vi "Current_Calib_Filenames.vi"(3 "Calib Filename":path[](array[path]), 4 "Channel Numbers":i16[](array[numeric]) min=0 max=7, 5 "Mode":T1) -> (0 "Calib Filename Out":path[](array[path]), 1 "Channel Numbers Out":i16[](array[numeric]) min=0 max=7)   [LabVIEW 2010]
uses:
  Controls/App_Global.ctl
  Globals/Constants_global.vi
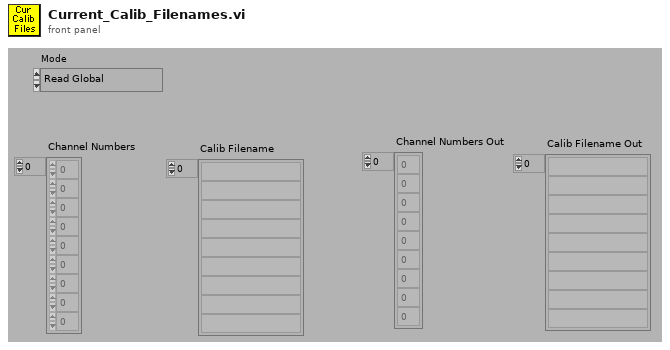
[diagram p1: front panel]
types:
  T1 = typedef "App_Global.ctl" = enum16{"Read Global", "Write to Global", "Initialise Array"}
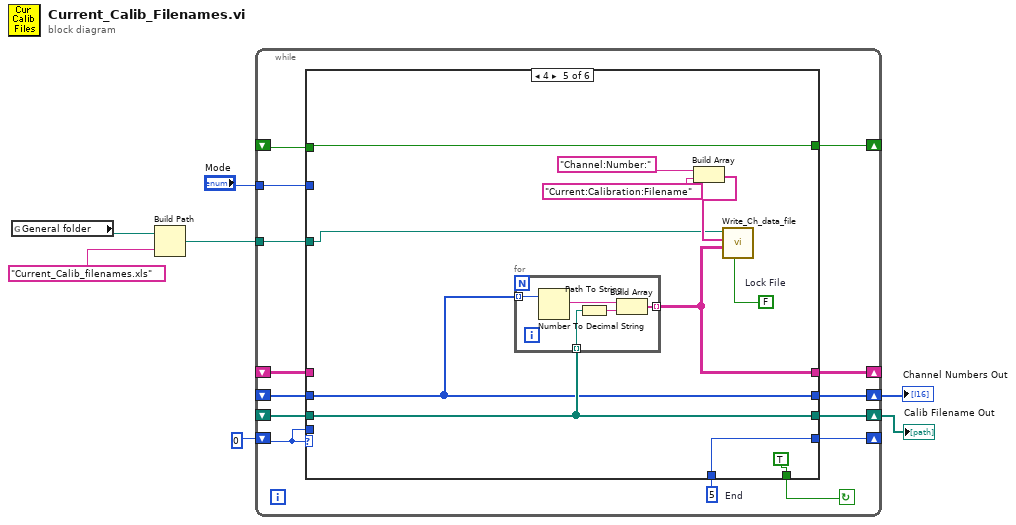
[diagram p0: block diagram]
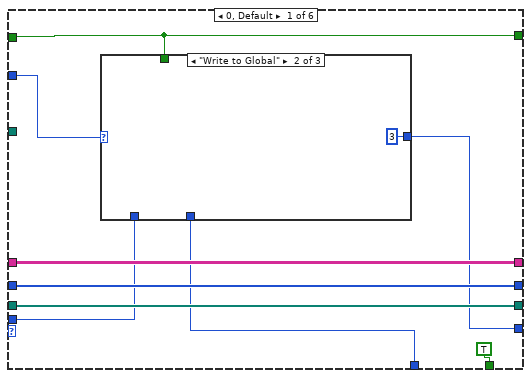
[diagram p2: hidden frame]
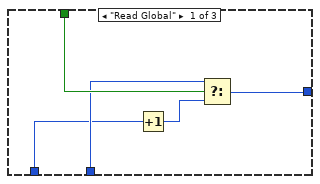
[diagram p3: hidden frame]
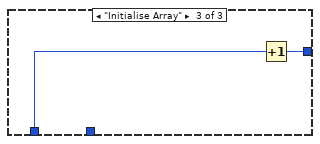
[diagram p4: hidden frame]
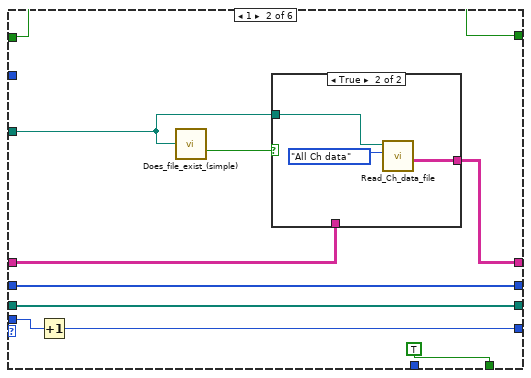
[diagram p5: hidden frame]
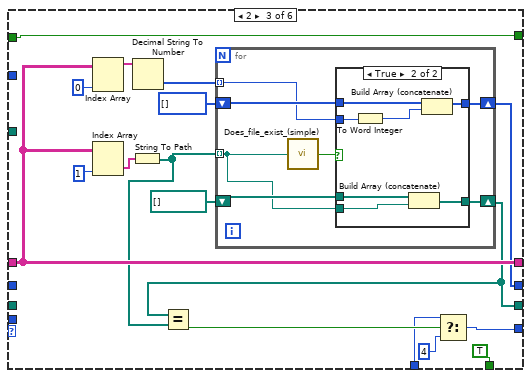
[diagram p7: hidden frame]
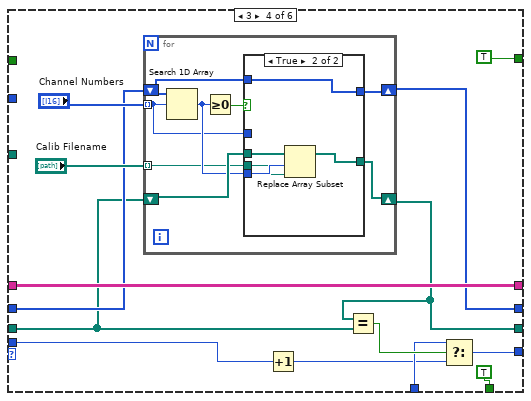
[diagram p9: hidden frame]
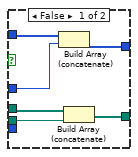
[diagram p10: hidden frame]
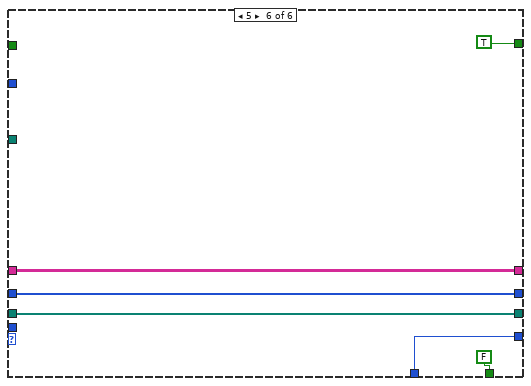
[diagram p11: hidden frame]
diagram:
  n1 = global read "Constants_global.vi" "General folder"() -> (w3:path)
  n2 = Build Path(base path=w3, name or relative path="Current_Calib_filenames.xls" ("Substring")) -> (appended path=w1:path)
  n3 = while {
    shift-left: _ -> [w10]
    shift-right: [w12] -> w4
    shift-left: _ -> [w11]
    shift-right: [w13] -> w5
    tunnel: "Mode" -> [w17]
    shift-left: 0 -> [w18]
    shift-right: [w19] -> _
    shift-left: _ -> [w14]
    shift-right: [w15] -> _
    shift-left: _ -> [w21]
    shift-right: [w16] -> _
    tunnel: w1 -> [w8]
    stop <- w20 continue-if-true
    w9 = 5  # End
    n4 = case shown="4" w18 {
      tunnel: w21 -> [w25 w45 w64 _ w129 _]
      tunnel: [TRUE TRUE TRUE TRUE TRUE FALSE] -> w20
      tunnel: [w22 w46 w55 w86 w128 w136] -> w19
      tunnel: w18 -> [w23 w47 _ w88 _ _]
      tunnel: w17 -> [w26 _ _ _ _ _]
      tunnel: [w25 w45 w64 TRUE w129 TRUE] -> w16
      tunnel: [w28 w43 w63 w98 w121 w139] -> w15
      tunnel: w14 -> [w28 w42 w63 w98 _ w139]
      tunnel: [w30 w41 w60 w93 w122 w138] -> w13
      tunnel: [w29 w40 w59 w92 w123 w137] -> w12
      tunnel: w11 -> [w30 w41 _ w94 w122 w138]
      tunnel: w10 -> [w29 w40 _ w91 w123 w137]
      tunnel: w9 -> [w24 _ w56 w89 w128 w136]
      tunnel: w8 -> [_ w39 _ _ w119 _]
      frame 0, Default {
        n5 = case shown="\"Write to Global\"" w26 {
          tunnel: w25 -> [w35 _ _]
          tunnel: w24 -> [w34 _ _]
          tunnel: w23 -> [w32 _ w38]
          tunnel: [w31 3 ("End") w37] -> w22
          frame "Read Global" {
            n6 = Increment(x=w32) -> (x+1=w33:i32)
            n7 = Select(t=w34, s=w35, f=w33) -> (s? t:f=w31:i32)
          }
          frame "Write to Global" {
          }
          frame "Initialise Array" {
            n8 = Increment(x=w38) -> (x+1=w37:i32)
          }
        }
      }
      frame 1 {
        n9 = Increment(x=w47) -> (x+1=w46:i32)
        n10 = call "Does_file_exist_(simple).vi"("Pathname"=w39) -> ("exists?"=w44:bool)
        n11 = case shown="True" w44 {
          tunnel: w39 -> [_ w51]
          tunnel: [w49 w50] -> w43
          tunnel: w42 -> [w49 _]
          frame False {
          }
          frame True {
            n12 = call "Read_Ch_data_file.vi"("Output"=enum16{"All Ch data", "The last few rows"}."All Ch data", "Filename"=w51) -> ("Channel Values"=w50:string[][])  [unwired: 3 in, 4 out]
          }
        }
      }
      frame 2 {
        n13 = Index Array(array=w63, index (col)=0 ("Index")) -> (element=w66:string[])  [unwired: 1 in]
        n14 = Index Array(array=w63, index (col)=1 ("Index")) -> (element=w65:string[])  [unwired: 1 in]
        n15 = String To Path(string=w65) -> (path=w58:path[])
        n16 = Decimal String To Number(string=w66) -> (number=w53:i32[])  [unwired: 3 out]
        n17 = for {
          shift-right: [w74] -> w60
          shift-right: [w71] -> w59
          shift-left: path[] [] -> [w72]
          tunnel: w58 -> [w70] mode=indexing
          shift-left: i16[] [] -> [w75]
          tunnel: w53 -> [w73] mode=indexing
          n18 = call "Does_file_exist_(simple).vi"("Pathname"=w70) -> ("exists?"=w76:bool)
          n19 = case shown="True" w76 {
            tunnel: w75 -> [w78 w85]
            tunnel: [w78 w84] -> w74
            tunnel: w73 -> [_ w80]
            tunnel: w72 -> [w77 w83]
            tunnel: [w77 w82] -> w71
            tunnel: w70 -> [_ w81]
            frame False {
            }
            frame True {
              n20 = To Word Integer(number=w80) -> (16bit integer=w79:i16)
              n21 = Build Array (concatenate)(w83, w81) -> (w82:path[])
              n22 = Build Array (concatenate)(w85, w79) -> (w84:i16[])
            }
          }
        }
        n23 = Equal?(x=w59, y=w58) -> (x = y?=w57:bool)
        n24 = Select(t=w56, s=w57, f=4) -> (s? t:f=w55:i32)
      }
      frame 3 {
        n25 = for {
          tunnel: "Channel Numbers" -> [w100] mode=indexing
          shift-right: [w103] -> w92
          shift-left: w91 -> [w106]
          tunnel: "Calib Filename" -> [w104] mode=indexing
          shift-right: [w102] -> w93
          shift-left: w94 -> [w101]
          n26 = Search 1D Array(1D array=w101, element=w100) -> (index of element=w105:i32)  [unwired: 1 out]
          n27 = Greater Or Equal To 0?(x=w105) -> (x >= 0?=w107:bool)
          n28 = case shown="True" w107 {
            tunnel: w106 -> [w110 w118]
            tunnel: w105 -> [_ w117]
            tunnel: w104 -> [w109 w116]
            tunnel: [w108 w115] -> w103
            tunnel: [w111 w114] -> w102
            tunnel: w101 -> [w113 w114]
            tunnel: w100 -> [w112 _]
            frame False {
              n29 = Build Array (concatenate)(w113, w112) -> (w111:i16[])
              n30 = Build Array (concatenate)(w110, w109) -> (w108:path[])
            }
            frame True {
              n31 = Replace Array Subset(array=w118, new element=w116, index=w117) -> (w115:path[])
            }
          }
        }
        n32 = Increment(x=w88) -> (x+1=w87:i32)
        n33 = Equal?(x=w92, y=w91) -> (x = y?=w90:bool)
        n34 = Select(t=w89, s=w90, f=w87) -> (s? t:f=w86:i32)
      }
      frame 4 {
        w120 = FALSE  # Lock File
        n35 = for {
          tunnel: w123 -> [w134] mode=indexing
          tunnel: w122 -> [w133] mode=indexing
          tunnel: [w131] -> w121 mode=indexing
          n36 = Number To Decimal String(number=w133) -> (decimal integer string=w132:string)  [unwired: 1 out]
          n37 = Path To String(path=w134) -> (string=w130:string)
          n38 = Build Array(w132, w130) -> (w131:string[])
        }
        n39 = Build Array("Channel:Number:", "Current:Calibration:Filename") -> (w124:string[])
        n40 = call "Write_Ch_data_file.vi"("Lock File"=w120, "Channel Values"=w121, "Channel names"=w124, "Filename"=w119) -> ()  [unwired: 4 in, 4 out]
      }
      frame 5 {
      }
    }
  }
  "Channel Numbers Out" <- w5
  "Calib Filename Out" <- w4
